vi "DAQmx Task Example_Configuration.vi"(7 "Rate (Hz)":dbl=1000.0 format="%0.2f", 8 "error in":errorcluster, 9 "Physical Strain Channel":string="Dev1/ai2", 10 "Physical TC Channel":string="Dev1/ai1", 11 "Physical Voltage Channel":string="Dev1/ai0") -> (0 "error out":errorcluster, 3 "task out":refnum<k21>)   [LabVIEW 2015]
doc: "This VI configures a task.\n\nYour program typically should execute this configuration code only once. To use this code in a loop, use the DAQmx ClearTask VI in the same loop."
uses:
  <vilib>/DAQmx/configure/trigger.llb/DAQmx Start Trigger (None).vi
  <vilib>/DAQmx/create/channels.llb/DAQmx Create Channel (AI-Voltage-Basic).vi
  <vilib>/DAQmx/configure/timing.llb/DAQmx Timing (Sample Clock).vi
panel:
  # "See Block Diagram for the steps below:\n1 - Create a DAQmx Task\n2 - Create a DAQmx Channel (Voltage) and add it to the task\n3 - Create a DAQmx Channel (Temperature) and add it to the task\n4 - Createa  DAQmx Channel (Strain) and add it to the task\n5 - Set up Task timing (continuous samples at 1000 Hz)\n6 - Set up Task triggering (none / SW trigger)\n7 - Export Task and Error info from SubVI"
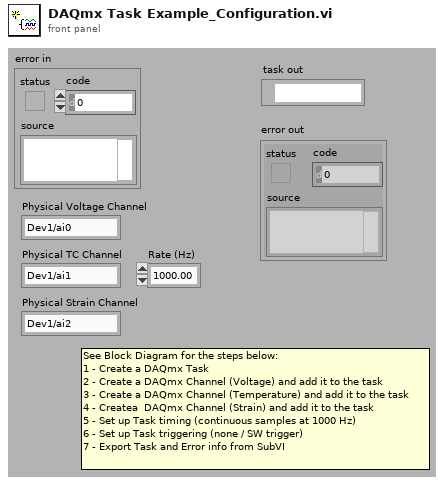
[diagram p1: front panel]
types:
  T1 = cluster{"strain configuration":i32, "lead resistance":dbl, "initial bridge voltage":dbl, "excitation source":i32, "excitation value":dbl}
  T2 = cluster{"gage factor":dbl, "nominal gage resistance":dbl, "poisson ratio":dbl}
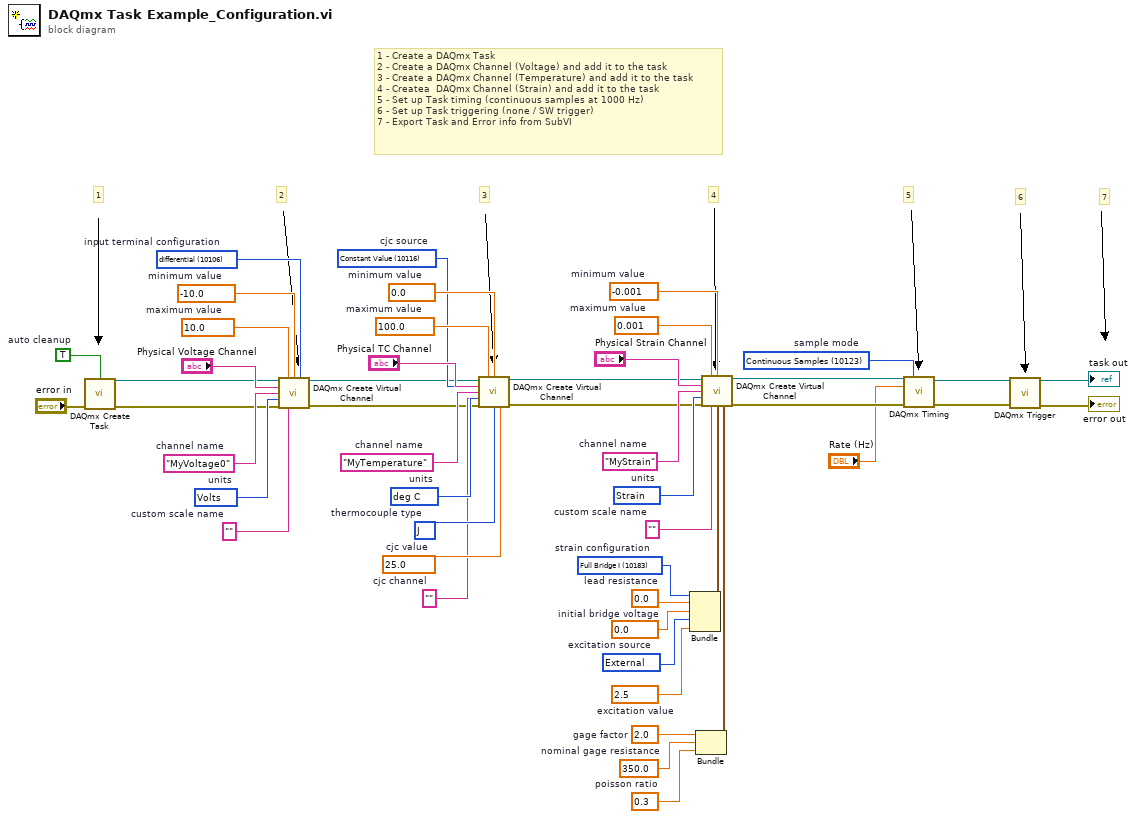
[diagram p0: block diagram]
diagram:
  w18 = 10106 items=["default"=-1, "differential"=10106, "RSE"=10083, "NRSE"=10078]  # input terminal configuration
  w17 = 10348 items=["Volts"=10348, "From Custom Scale"=10065]  # units
  w16 = "MyVoltage0"  # channel name
  w15 = ""  # custom scale name
  w14 = -10.0  # minimum value
  w13 = 10.0  # maximum value
  w25 = 0.0  # lead resistance
  w28 = 0.3  # poisson ratio
  w24 = 0.0  # initial bridge voltage
  w29 = 350.0  # nominal gage resistance
  w27 = 2.0  # gage factor
  w22 = 2.5  # excitation value
  w23 = 10167 items=["Internal"=10200, "External"=10167, "None"=10230]  # excitation source
  w26 = 10183 items=["Full Bridge I"=10183, "Full Bridge II"=10184, "Full Bridge III"=10185, "Half Bridge I"=10188, "Half Bridge II"=10189, "Quarter Bridge I"=10271, "Quarter Bridge II"=10272]  # strain configuration
  w31 = 10299 items=["Strain"=10299, "From Custom Scale"=10065]  # units
  w32 = "MyStrain"  # channel name
  w33 = ""  # custom scale name
  w34 = -0.001  # minimum value
  w35 = 0.001  # maximum value
  w38 = ""  # cjc channel
  w39 = u32 10116 items=["Internal"=10200, "Constant Value"=10116, "Channel"=10113]  # cjc source
  w40 = 25.0  # cjc value
  w41 = 10072 items=["J"=10072, "K"=10073, "N"=10077, "R"=10082, "S"=10085, "T"=10086, "B"=10047, "E"=10055]  # thermocouple type
  w42 = 10143 items=["deg C"=10143, "deg F"=10144, "Kelvins"=10325, "deg R"=10145, "From Custom Scale"=10065]  # units
  w37 = "MyTemperature"  # channel name
  w43 = 0.0  # minimum value
  w44 = 100.0  # maximum value
  w46 = 10123 items=["Finite Samples"=10178, "Continuous Samples"=10123]  # sample mode
  w47 = TRUE  # auto cleanup
  # "7"
  # "1 - Create a DAQmx Task\n2 - Create a DAQmx Channel (Voltage) and add it to the task\n3 - Create a DAQmx Channel (Temperature) and add it to the task\n4 - Createa  DAQmx Channel (Strain) and add it to the task\n5 - Set up Task timing (continuous samples at 1000 Hz)\n6 - Set up Task triggering (none / SW trigger)\n7 - Export Task and Error info from SubVI"
  # "6"
  # "5"
  # "4"
  # "3"
  # "2"
  # "1"
  n1 = call <vilib>:"DAQmx Create Task.vi"("auto cleanup"=w47, "error in"="error in") -> ("task out"=w9:refnum<k21>, "error out"=w8:errorcluster)  [unwired: 12 in]
  n2 = call-poly <vilib>:"DAQmx Create Virtual Channel.vi"("task in"=w9, "maximum value"=w13, "minimum value"=w14, "input terminal configuration"=w18, "physical channels"="Physical Voltage Channel", "name to assign"=w16, "units"=w17, "error in"=w8, "custom scale name"=w15) -> ("task out"=w11:refnum<k21>, "error out"=w10:errorcluster)  [unwired: 5 in]
  n3 = call-poly <vilib>:"DAQmx Create Virtual Channel.vi"("task in"=w11, "maximum value"=w44, "minimum value"=w43, "physical channels"="Physical TC Channel", 6:w39, "name to assign"=w37, "units"=w42, 10:w38, "error in"=w10, 13:w41, 14:w40) -> ("task out"=w20:refnum<k21>, "error out"=w19:errorcluster)  [unwired: 3 in]
  n4 = Bundle("strain configuration"=w26, "lead resistance"=w25, "initial bridge voltage"=w24, "excitation source"=w23, "excitation value"=w22) -> (w21:T1)  [unwired: 1 in]
  n5 = Bundle("gage factor"=w27, "nominal gage resistance"=w29, "poisson ratio"=w28) -> (w30:T2)  [unwired: 1 in]
  n6 = call-poly <vilib>:"DAQmx Create Virtual Channel.vi"("task in"=w20, "maximum value"=w35, "minimum value"=w34, "physical channels"="Physical Strain Channel", "name to assign"=w32, "units"=w31, "error in"=w19, "custom scale name"=w33, 13:w21, 14:w30) -> ("task out"=w7:refnum<k21>, "error out"=w6:errorcluster)  [unwired: 4 in]
  n7 = call-poly <vilib>:"DAQmx Timing.vi"("task/channels in"=w7, "sample mode"=w46, "rate"="Rate (Hz)", "error in"=w6) -> ("task out"=w5:refnum<k21>, "error out"=w4:errorcluster)  [unwired: 10 in]
  n8 = call-poly <vilib>:"DAQmx Trigger.vi"("task/channels in"=w5, "error in"=w4) -> ("task out"=→"task out":refnum<k21>, "error out"=→"error out":errorcluster)  [unwired: 12 in]
